vi "Server_Data Log.vi"(8 "error in":errorcluster, 11 "Data File Format":T1) -> (0 "error out":errorcluster)   [LabVIEW 2018, in "Cloud Server.lvlib"]
uses:
  Cloud Server.lvlib
  Com VIs/Data Def/Data File Format.ctl
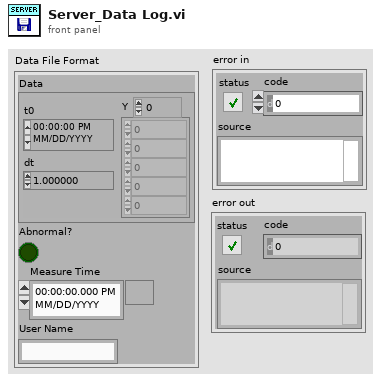
[diagram p1: front panel]
types:
  T1 = typedef "Data File Format.ctl" = cluster{"Data":waveform(dbl), "Abnormal?":bool, "Measure Time":timestamp, "User Name":string}
  T2 = enum16{"open", "replace", "create", "open or create", "replace or create", "replace or create with confirmation"}
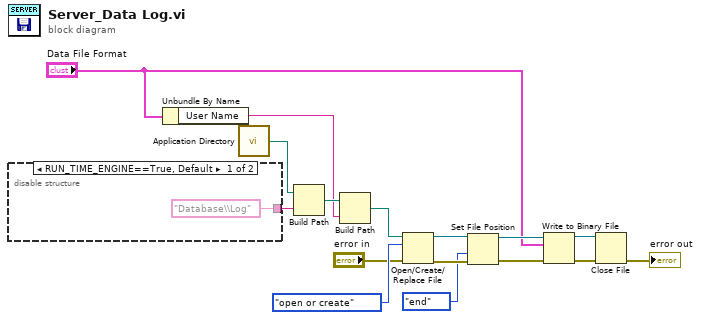
[diagram p0: block diagram]
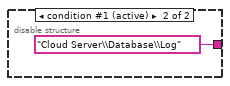
[diagram p2: hidden frame]
diagram:
  n1 = disable-structure shown="RUN_TIME_ENGINE==True, Default" {
    disable-tunnel: ["Database\\Log" ("name or relative path") "Cloud Server\\Database\\Log" ("name or relative path")] -> w16
    frame condition #0 {
    }
    frame condition #1 (active) {
    }
  }
  n2 = Unbundle By Name("Data File Format") -> ("User Name"=w13:string)
  n3 = call <vilib>:"Application Directory.vi"() -> ("Application Directory"=w15:path)
  n4 = Build Path(base path=w15, name or relative path=w16) -> (appended path=w14:path)
  n5 = Build Path(base path=w14, name or relative path=w13) -> (appended path=w12:path)
  n6 = Open/Create/Replace File(file path (use dialog)=w12, error in="error in", operation (0:open)=T2."open or create") -> (refnum out=w6:refnum<file>, error out=w3:errorcluster)  [unwired: 3 in, 1 out]
  n7 = Set File Position(refnum=w6, from (0:start)=enum16{"start", "end", "current"}."end", error in=w3) -> (refnum out=w5:refnum<file>, error out=w4:errorcluster)  [unwired: 1 in]
  n8 = Write to Binary File(file (use dialog)=w5, data="Data File Format", error in=w4) -> (refnum out=w8:refnum<file>, error out=w9:errorcluster)  [unwired: 3 in, 1 out]
  n9 = Close File(refnum=w8, error in=w9) -> (error out=→"error out":errorcluster)  [unwired: 1 out]
